vi "Configure Output Limits.vi"(0 "VISA resource name":refnum<visa-resource-name>, 1 "AC Voltage Limit (10.000 V)":dbl=10.0 format="%.3g", 5 "AC Current Limit (5.000 A)":dbl=5.0 format="%.3g", 7 "DC Positive Voltage Limit (424.000 V)":dbl=424.0 format="%.1f", 9 "DC Negative Voltage Limit (-424.000 V)":dbl=-424.0 min=-424.0 max=0.0 format="%.1f", 11 "error in (no error)":errorcluster, 12 "Power Limit (2000 VA)":dbl=2000.0 format="%.2f", 13 "Current Limit Delay (0 ms)":u32) -> (4 "VISA resource name out":refnum<visa-resource-name>, 15 "error out":errorcluster)   [LabVIEW 2018, in "BK Precision 983X Series.lvlib"]
doc: "Configures the AC and DC voltage limits, current limit, power limit, and the current limit delay time."
uses:
  <instrlib>/BK Precision 983X Series/BK Precision 983X Series.lvlib
panel:
  # "V"
  # "VA"
  # "A"
  # "V"
  # "V"
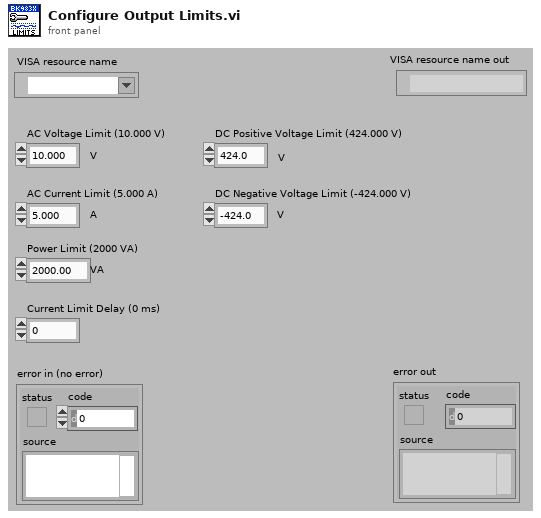
[diagram p1: front panel]
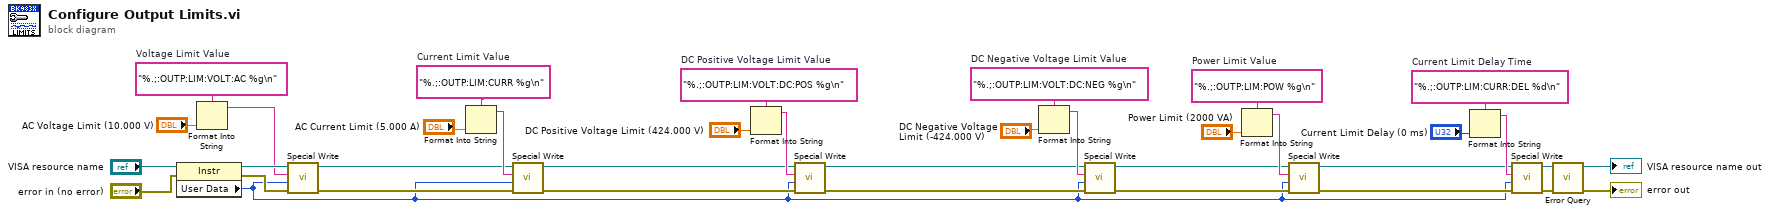
[diagram p0: block diagram]
diagram:
  w26 = "%.;:OUTP:LIM:CURR:DEL %d\n"  # Current Limit Delay Time
  w27 = "%.;:OUTP:LIM:POW %g\n"  # Power Limit Value
  w31 = "%.;:OUTP:LIM:VOLT:DC:NEG %g\n"  # DC Negative Voltage Limit Value
  w32 = "%.;:OUTP:LIM:VOLT:DC:POS %g\n"  # DC Positive Voltage Limit Value
  w33 = "%.;:OUTP:LIM:CURR %g\n"  # Current Limit Value
  w35 = "%.;:OUTP:LIM:VOLT:AC %g\n"  # Voltage Limit Value
  n1 = property class="Instr"(reference="VISA resource name", error in="error in (no error)") -> (reference out=w21:refnum<visa-resource-name>, error out=w20:errorcluster, "User Data"=w1:u32)
  n2 = Format Into String(format string=w35, "AC Voltage Limit (10.000 V)") -> (resulting string=w19:string)  [unwired: 2 in, 1 out]
  n3 = call <instrlib>:"Special Write.vi"("error in (no error)"=w20, "Delay (0 ms)"=w1, "Input String"=w19, "VISA resource name"=w21) -> ("error out"=w2:errorcluster, "VISA resource name out"=w17:refnum<visa-resource-name>)  [unwired: 6 in]
  n4 = Format Into String(format string=w33, "AC Current Limit (5.000 A)") -> (resulting string=w18:string)  [unwired: 2 in, 1 out]
  n5 = call <instrlib>:"Special Write.vi"("error in (no error)"=w2, "Delay (0 ms)"=w1, "Input String"=w18, "VISA resource name"=w17) -> ("error out"=w3:errorcluster, "VISA resource name out"=w15:refnum<visa-resource-name>)  [unwired: 6 in]
  n6 = Format Into String(format string=w32, "DC Positive Voltage Limit (424.000 V)") -> (resulting string=w16:string)  [unwired: 2 in, 1 out]
  n7 = call <instrlib>:"Special Write.vi"("error in (no error)"=w3, "Delay (0 ms)"=w1, "Input String"=w16, "VISA resource name"=w15) -> ("error out"=w4:errorcluster, "VISA resource name out"=w13:refnum<visa-resource-name>)  [unwired: 6 in]
  n8 = Format Into String(format string=w31, "DC Negative Voltage Limit (-424.000 V)") -> (resulting string=w14:string)  [unwired: 2 in, 1 out]
  n9 = call <instrlib>:"Special Write.vi"("error in (no error)"=w4, "Delay (0 ms)"=w1, "Input String"=w14, "VISA resource name"=w13) -> ("error out"=w5:errorcluster, "VISA resource name out"=w11:refnum<visa-resource-name>)  [unwired: 6 in]
  n10 = Format Into String(format string=w27, "Power Limit (2000 VA)") -> (resulting string=w12:string)  [unwired: 2 in, 1 out]
  n11 = call <instrlib>:"Special Write.vi"("error in (no error)"=w5, "Delay (0 ms)"=w1, "Input String"=w12, "VISA resource name"=w11) -> ("error out"=w6:errorcluster, "VISA resource name out"=w9:refnum<visa-resource-name>)  [unwired: 6 in]
  n12 = Format Into String(format string=w26, "Current Limit Delay (0 ms)") -> (resulting string=w10:string)  [unwired: 2 in, 1 out]
  n13 = call <instrlib>:"Special Write.vi"("error in (no error)"=w6, "Delay (0 ms)"=w1, "Input String"=w10, "VISA resource name"=w9) -> ("error out"=w7:errorcluster, "VISA resource name out"=w8:refnum<visa-resource-name>)  [unwired: 6 in]
  n14 = call <instrlib>:"Error Query.vi"("error in (no error)"=w7, "VISA resource name"=w8) -> ("error out"=→"error out":errorcluster, "VISA resource name out"=→"VISA resource name out":refnum<visa-resource-name>)  [unwired: 6 in, 2 out]
